vi "Init_Serial.vi"(8 "error in (no error)":errorcluster, 10 "Board":u8, 11 "session in":refnum<k35>) -> (0 "error out":errorcluster, 3 "session out":refnum<k35>)   [LabVIEW 2021]
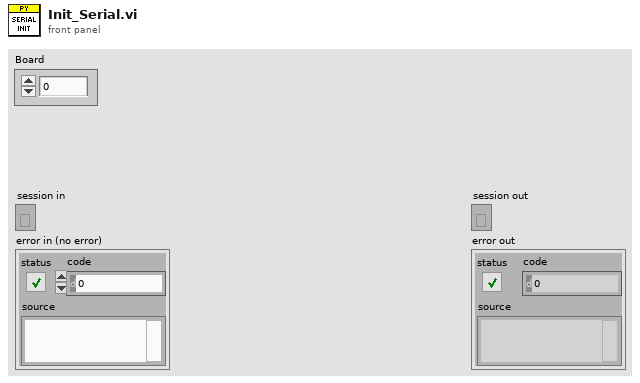
[diagram p1: front panel]
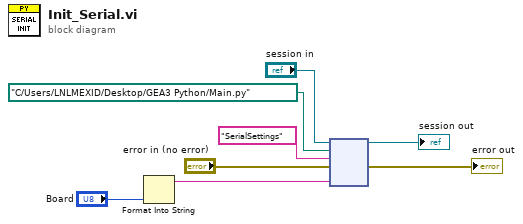
[diagram p0: block diagram]
diagram:
  n1 = Format Into String("Board") -> (resulting string=w1:string)  [unwired: 3 in, 1 out]
  n2 = node("session in", path "C:/Users/LNLMEXID/Desktop/GEA3 Python/Main.py" ("module path"), "SerialSettings" ("function name"), "error in (no error)", w1) -> (→"session out":refnum<k35>, →"error out":errorcluster)  [unwired: 3 in, 2 out]
